vi "test_scale_calculation.vi"() -> ()   [LabVIEW 2019]
panel:
  out "mm/pix":sgl
  out "Error Out":errorcluster
  in  "mm":sgl
  out "Image":T1(plugin-control)
  in  "File Path":path
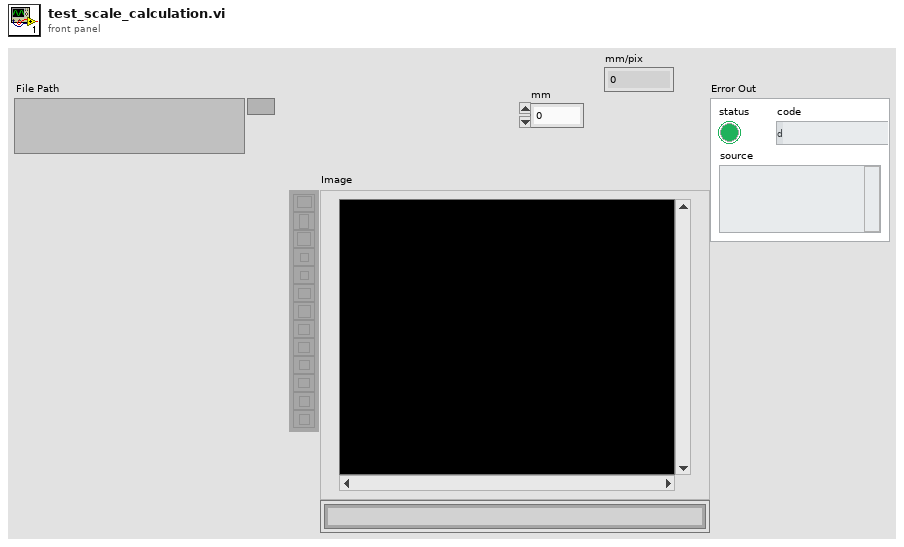
[diagram p1: front panel]
types:
  T1 = typedef "IMAQ Image.ctl" = refnum<image>
  T2 = cluster{"Global Rectangle":i32[], "Contours":cluster{"Contour Type":u32, "ROI Type":u32, "Points":i32[]}[]}
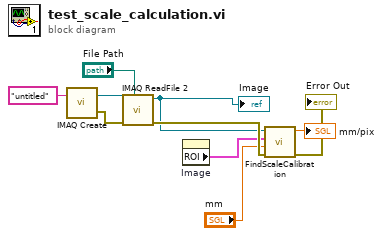
[diagram p0: block diagram]
diagram:
  n1 = call "IMAQ Create"("Image Name"="untitled") -> ("New Image"=w9:T1, "error out"=w7:errorcluster)  [unwired: 4 in]
  n2 = call "IMAQ ReadFile 2"("File Path"="File Path", "error in (no error)"=w7, "Image"=w9) -> ("error out"=w6:errorcluster, "Image Out"=w5:T1)  [unwired: 4 in, 3 out]
  "Image" <- w5
  n3 = property on="Image" class="ImageControl"() -> ("ROI"=w4:T2)  [unwired: 2 in, 2 out]
  n4 = call "FindScaleCalibration.vi"("Error In"=w6, "mm"="mm", "ROI Descriptor"=w4, "Image Src"=w5) -> ("Error Out"=→"Error Out":errorcluster, "mm/pix"=→"mm/pix":sgl)  [unwired: 6 in]
